vi "ROI group-Delete ROI group.vi"(8 "error in (no error)":errorcluster, 9 "Dialogue message type":enum16{"Warning", "Attention"}(ring), 11 "Save? (T)":bool=TRUE) -> ()   [LabVIEW 2020]
uses:
  Experiment header interface/Typedefs/Save-Load-Save as-Load last enum.ctl
  Global variables/gl_Functional Imaging-Global variables.vi
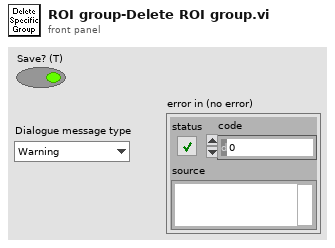
[diagram p1: front panel]
types:
  T1 = typedef "Save-Load-Save as-Load last enum.ctl" = enum16{"Save file", "Save file as", "Load file", "Load last file"}
  T2 = typedef "Functional Imging UI Refs.ctl" = cluster{"Menu ref":refnum<k9>, "Image control":refnum<vi>, "VI ref":refnum<vi>, "XGrapher":refnum<vi>, "Smoothing":refnum<vi>, "POI Averaging":refnum<vi>, "Normalize":refnum<vi>, "POI data points in each trial":refnum<vi>, "Channel":refnum<vi>, "Experiment data folder path":refnum<vi>, "[ROI vis]":refnum<vi>, "[Groups] visbl":T3, "Group Name":refnum<vi>, "POI index":refnum<vi>, "Trial No.":refnum<vi>, "Intensity Zoom":refnum<vi>, "Trial Cursor Enabled":refnum<vi>, "Number of Trials (ind 1)":refnum<vi>, "Number of Trials (ind 2)":refnum<vi>, "MiniScans Available":refnum<vi>, "POI Available":refnum<vi>, "Defer graph updates":refnum<vi>, "Waveform selector":refnum<vi>, "#of selected POI":refnum<vi>, "#of selected MiniScans":refnum<vi>, "#of selected groups":refnum<vi>, "Max Z-Projection":refnum<vi>, "Z-Plane Selector":refnum<vi>, "Index of miniscan point to visualise":refnum<vi>, "ROI vis. mode":refnum<vi>, "Total # of points":refnum<vi>, "Index of group clicked on":refnum<vi>, "Pane 1":refnum<vi>, "Pane 2":refnum<vi>, "Pane 3":refnum<vi>, "Pane 4":refnum<vi>, "Pane 5":refnum<vi>, "Pane 6":refnum<vi>, "Deselect all ROI":refnum<vi>, "Deselect all groups":refnum<vi>}
  T3 = typedef "Groups array referecne.ctl" = refnum<vi>
  T4 = typedef "Group sel cluster.ctl" = cluster{"Group number":string, "Group Name":string, "Visibility":bool, "Highlight":bool}
  T5 = typedef "ROI group info cluster.ctl" = cluster{"Group name":string, "# ROI in group":i32, "ROI numbers in group":i32[], "Group region specifier cluster":T6}
  T6 = typedef "ROI Descriptor" = cluster{"Global Rectangle":i32[], "Contours":cluster{"ID":enum32{"External", "Internal"}, "Type":u32, "Coordinates":i32[]}[]}
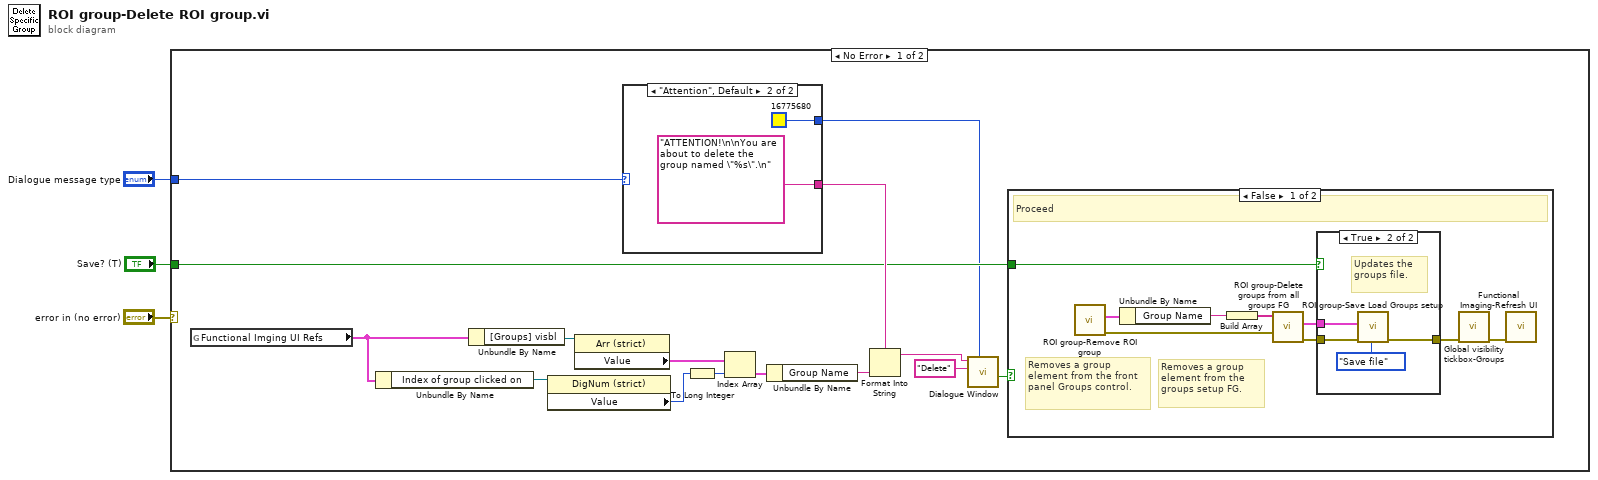
[diagram p0: block diagram]
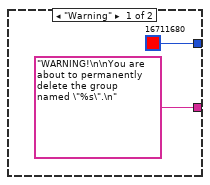
[diagram p2: hidden frame]
diagram:
  n1 = case shown="No Error" "error in (no error)" {
    tunnel: "Save? (T)" -> [w6 _]
    tunnel: "Dialogue message type" -> [w5 _]
    frame No Error {
      n2 = global read "gl_Functional Imaging-Global variables.vi" "Functional Imging UI Refs"() -> (w12:T2)
      n3 = Unbundle By Name(w12) -> ("Index of group clicked on"=w11:refnum<vi>)
      n4 = Unbundle By Name(w12) -> ("[Groups] visbl"=w10:T3)
      n5 = property on="Property Node" class="DigNum (strict)"(reference=w11) -> ("Value"=w14:i16)  [unwired: 1 in, 2 out]
      n6 = property on="Property Node" class="Arr (strict)"(reference=w10) -> ("Value"=w13:T4[])  [unwired: 1 in, 2 out]
      n7 = case shown="\"Attention\", Default" w5 {
        tunnel: ["WARNING!\n\nYou are about to permanently delete the group named \"%s\".\n" ("Message string") "ATTENTION!\n\nYou are about to delete the group named \"%s\".\n" ("Message string")] -> w8
        tunnel: [u32 16711680 ("Colour") u32 16775680 ("Colour")] -> w4
        frame "Warning" {
        }
        frame "Attention", Default {
        }
      }
      n8 = To Long Integer(number=w14) -> (32bit integer=w15:i32)
      n9 = Index Array(array=w13, index=w15) -> (element=w16:T4)
      n10 = Unbundle By Name(w16) -> ("Group Name"=w9:string)
      n11 = Format Into String(format string=w8, w9) -> (resulting string=w7:string)  [unwired: 2 in, 1 out]
      n12 = call "Dialogue Window.vi"("Colour"=w4, "Caption-Right button (OK)"="Delete", "Message string"=w7) -> ("Cancelled (Left button pressed)"=w18:bool)  [unwired: 6 in, 2 out]
      n13 = case shown="False" w18 {
        tunnel: w6 -> [w25 _]
        frame False {
          # "Removes a group element from the groups setup FG."
          # "Removes a group element from the front panel Groups control."
          # "Proceed"
          n14 = call "ROI group-Remove ROI group.vi"() -> ("error out"=w29:errorcluster, "Deleted group setup"=w30:T4)  [unwired: 10 in]
          n15 = Unbundle By Name(w30) -> ("Group Name"=w28:string)
          n16 = Build Array(w28) -> (w31:string[])
          n17 = call "ROI group-Delete groups from all groups FG.vi"("error in (no error)"=w29, "Names of groups to delete"=w31) -> ("error out"=w27:errorcluster, "Updated groups setup"=w26:T5[])  [unwired: 8 in]
          n18 = case shown="True" w25 {
            tunnel: w27 -> [w32 w35]
            tunnel: w26 -> [_ w34]
            tunnel: [w32 w33] -> w23
            frame False {
            }
            frame True {
              # "Updates the groups file."
              n19 = call "ROI group-Save Load Groups setup.vi"("error in (no error)"=w35, "Function"=Save-Load-Save_as-Load_last_enum."Save file", "Groups setup to save"=w34) -> ("error out"=w33:errorcluster)  [unwired: 7 in, 1 out]
            }
          }
          n20 = call "Global visibility tickbox-Groups.vi"("error in (no error)"=w23) -> ("error out"=w24:errorcluster)  [unwired: 10 in]
          n21 = call "Functional Imaging-Refresh UI.vi"("error in (no error)"=w24) -> ()  [unwired: 11 in]
        }
        frame True {
          # "Cancelled"
        }
      }
    }
    frame Error {
    }
  }
